vi "AddArguments.vi"(6 "inputs":T1[](array[typedef]), 7 "parser name":string="parser", 8 "error in":errorcluster, 11 "VI Interpreter in":refnum<class "VI Interpreter.lvclass">) -> (0 "error out":errorcluster, 3 "VI Interpreter out":refnum<class "VI Interpreter.lvclass">, 4 "names":string[](array[string]), 5 "arguments":string[](array[string]))   [LabVIEW 2014, in "Raspberry Pi Compatible Compiler for LabVIEW.lvlib" / "PyConvBD.lvclass"]
uses:
  PyConvBD.lvclass
  VI Interpreter/Classes/VI Interpreter/VI Interpreter.lvclass
  TypeDefs/ConsoleArg_TD.ctl
  Parsing/Python Functions.lvlib
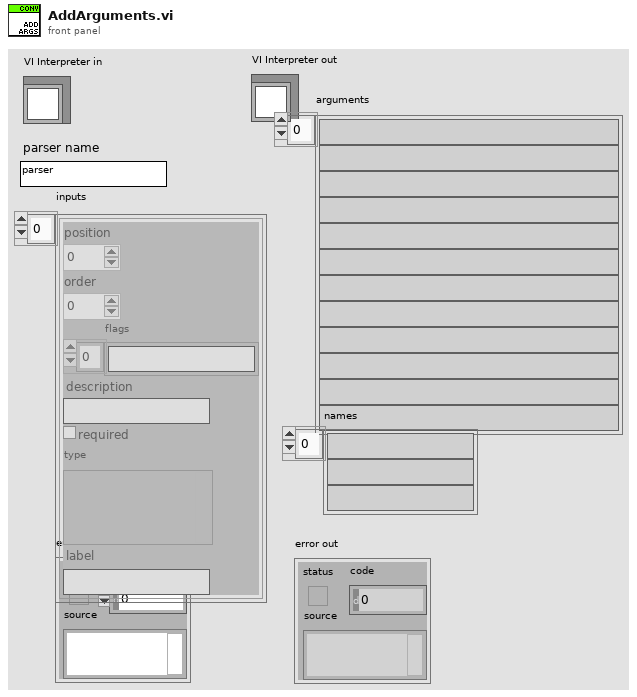
[diagram p1: front panel]
types:
  T1 = typedef "Raspberry Pi Compatible Compiler for LabVIEW.lvlib/PyConvBD.lvclass/ConsoleArg_TD.ctl" = cluster{"position":i32, "order":i32, "flags":string[], "description":string, "required":bool, "type":variant, "label":string}
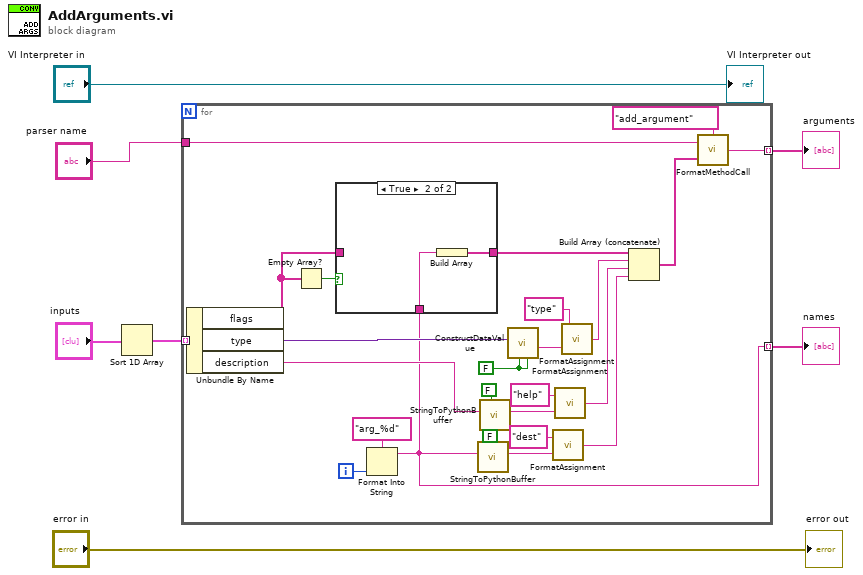
[diagram p0: block diagram]
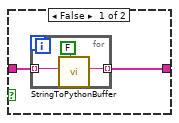
[diagram p2: hidden frame]
diagram:
  n1 = Sort 1D Array(array="inputs") -> (sorted array=w6:T1[])
  n2 = for {
    tunnel: w6 -> [w27] mode=indexing
    tunnel: "parser name" -> [w31]
    tunnel: [w21] -> w4 mode=indexing
    tunnel: [w8] -> w1 mode=indexing
    i -> [w14]
    w29 = FALSE ("value")
    n3 = Unbundle By Name(w27) -> ("flags"=w17:string[], "type"=w26:variant, "description"=w22:string)
    n4 = Empty Array?(array=w17) -> (empty?=w18:bool)
    n5 = Format Into String(format string="arg_%d", w14) -> (resulting string=w8:string)  [unwired: 2 in, 1 out]
    n6 = case shown="True" w18 {
      tunnel: w17 -> [w33 _]
      tunnel: [w34 w39] -> w16
      tunnel: w8 -> [_ w38]
      frame False {
        n7 = for {
          tunnel: w33 -> [w36] mode=indexing
          tunnel: [w35] -> w34 mode=indexing
          n8 = call "StringToPythonBuffer.vi"("Buffer"=FALSE, "string"=w36) -> ("python string"=w35:string)  [unwired: 7 in]
        }
      }
      frame True {
        n9 = Build Array(w38) -> (w39:string[])
      }
    }
    n10 = call "StringToPythonBuffer.vi"("Buffer"=FALSE, "string"=w8) -> ("python string"=w10:string)  [unwired: 7 in]
    n11 = call "StringToPythonBuffer.vi"("Buffer"=FALSE, "string"=w22) -> ("python string"=w24:string)  [unwired: 7 in]
    n12 = call "ConstructDataValue.vi"("label"=w29, "value"=w29, "Value"=w26) -> ("type"=w30:string)  [unwired: 5 in, 1 out]
    n13 = call "FormatAssignment.vi"("value"=w10, "name"="dest") -> ("python assignment"=w9:string)
    n14 = call "FormatAssignment.vi"("value"=w24, "name"="help") -> ("python assignment"=w11:string)
    n15 = call "FormatAssignment.vi"("value"=w30, "name"="type") -> ("python assignment"=w20:string)
    n16 = Build Array (concatenate)(w16, w20, w11, w9) -> (w19:string[])
    n17 = call "FormatMethodCall.vi"("method"="add_argument", "parameters"=w19, "object"=w31) -> ("python object"=w21:string)
  }
  "arguments" <- w4
  "names" <- w1
  "error out" <- "error in"
  "VI Interpreter out" <- "VI Interpreter in"
